vi "Hide Panel.vi"(8 "error in (no error)":errorcluster, 11 "View In":refnum<class "View.lvclass">) -> (0 "error out":errorcluster, 3 "View Out":refnum<class "View.lvclass">)   [LabVIEW 2020, in "View.lvclass"]
doc: "Hide the front panel of the View."
uses:
  View.lvclass
  C:/Users/anton/Documents/GitHub/Triarc-Framework/source/Framework/Process/Process.lvclass
  Process/Process.lvclass/Process.ctl
  View.lvclass/View.ctl
  Process/Public/Get Lifecycle State.vi
  Process/Protected/Messaging/Request Message.vi
  <vilib>/AdvancedString/1D String Array to Delimited String.vi
  Process/Private/SubVIs/Enqueue Request Message.vi
  <vilib>/Utility/error.llb/Error Cluster From Error Code.vi
  Process/Private/SubVIs/Wait for Response Message.vi
  Process/Process.lvclass
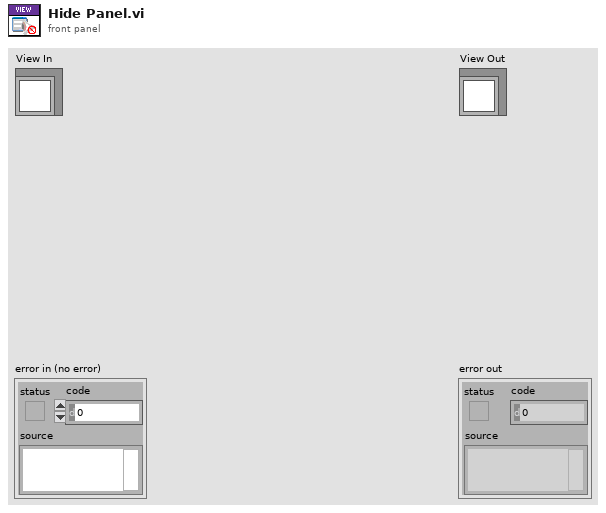
[diagram p1: front panel]
types:
  T1 = typedef "Process.lvclass/Access Mode.ctl" = enum16{"Read", "Request"}
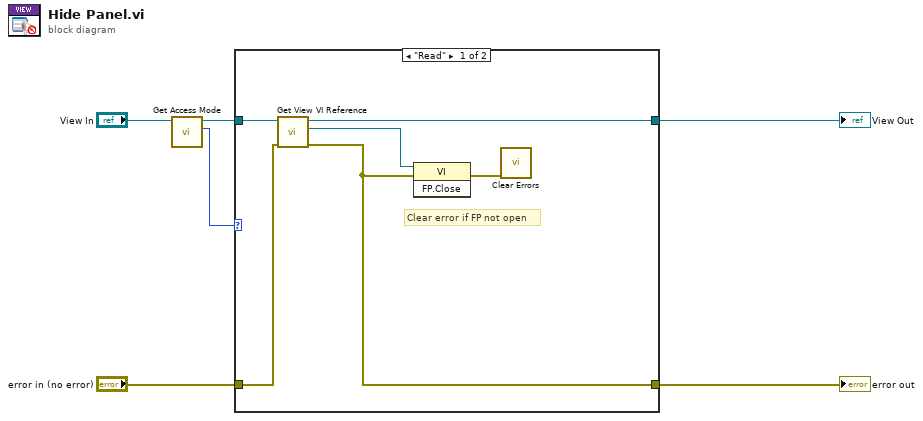
[diagram p0: block diagram]
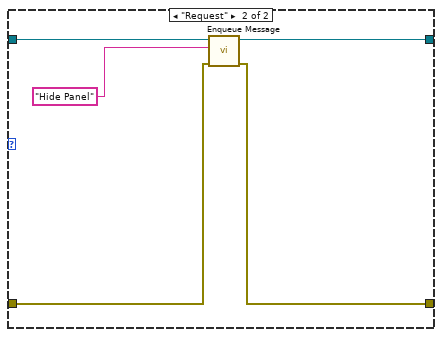
[diagram p2: hidden frame]
diagram:
  n1 = call "Get Access Mode.vi"("Process In"="View In") -> ("Access Mode"=w1:T1, "Process Out"=w2:refnum<class "View.lvclass">)  [unwired: 8 in, 1 out]
  n2 = case shown="\"Read\"" w1 {
    tunnel: [w10 w17] -> w5
    tunnel: [w7 w16] -> w4
    tunnel: "error in (no error)" -> [w9 w15]
    tunnel: w2 -> [w11 w13]
    frame "Read" {
      # "Clear error if FP not open"
      n3 = call "Get View VI Reference.vi"("error in (no error)"=w9, "UI View In"=w11) -> ("error out"=w7:errorcluster, "View VI Reference"=w12:refnum<vi>, "UI View Out"=w10:refnum<class "View.lvclass">)  [unwired: 7 in]
      n4 = invoke class="VI" method="FP.Close"(reference=w12, error in=w7) -> (error out=w8:errorcluster)  [unwired: 1 in, 2 out]
      n5 = call <vilib>:"Clear Errors.vi"("error in (no error)"=w8) -> ()  [unwired: 5 in, 2 out]
    }
    frame "Request" {
      n6 = call "Enqueue Message.vi"("error in (no error)"=w15, "Message"="Hide Panel", "Process In"=w13) -> ("error out"=w16:errorcluster, "Process Out"=w17:refnum<class "View.lvclass">)  [unwired: 7 in]
    }
  }
  "error out" <- w4
  "View Out" <- w5
